vi "Read Roles.vi"(8 "error in (no error)":errorcluster, 11 "TimeoutPlay in":refnum<class "TimeoutPlay.lvclass">) -> (0 "error out":errorcluster, 2 "Roles":T1, 3 "TimeoutPlay out":refnum<class "TimeoutPlay.lvclass">)   [LabVIEW 2023, in "TimeoutPlay.lvclass"]
uses:
  TimeoutPlay.lvclass
  TimeoutRole_class/TimeoutRole.lvclass
  TimeoutPlay.lvclass/TimeoutPlay.ctl
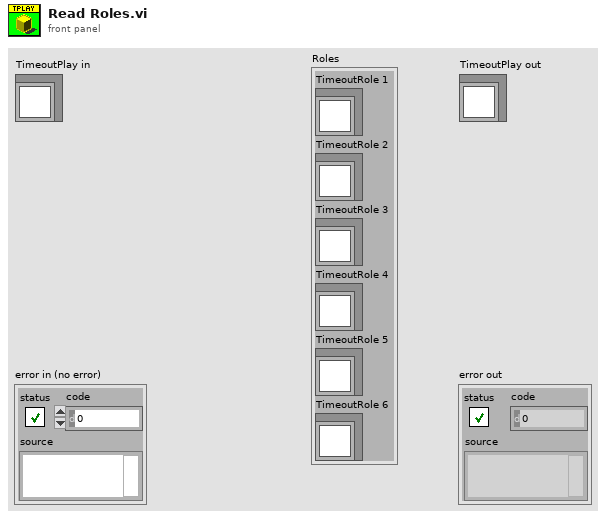
[diagram p1: front panel]
types:
  T1 = cluster{"TimeoutRole 1":refnum<class "TimeoutRole.lvclass">, "TimeoutRole 2":refnum<class "TimeoutRole.lvclass">, "TimeoutRole 3":refnum<class "TimeoutRole.lvclass">, "TimeoutRole 4":refnum<class "TimeoutRole.lvclass">, "TimeoutRole 5":refnum<class "TimeoutRole.lvclass">, "TimeoutRole 6":refnum<class "TimeoutRole.lvclass">}
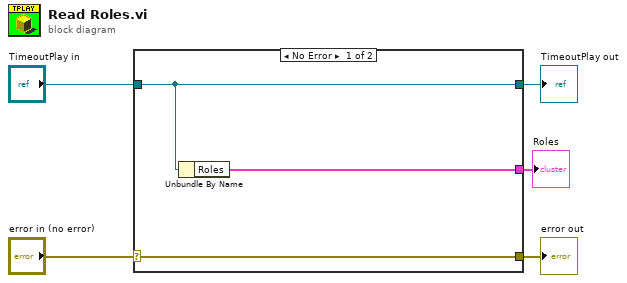
[diagram p0: block diagram]
diagram:
  n1 = case shown="No Error" "error in (no error)" {
    selector: "error in (no error)" -> [w8 w9]
    tunnel: [w8 w9] -> w4
    tunnel: [w7 w10] -> w2
    tunnel: "TimeoutPlay in" -> [w7 w10]
    tunnel: [w6 _] -> w1
    frame No Error {
      n2 = Unbundle By Name(w7) -> ("Roles"=w6:T1)
    }
    frame Error {
    }
  }
  "error out" <- w4
  "TimeoutPlay out" <- w2
  "Roles" <- w1
